vi "Counter - Read Encoder.vi"() -> ()   [LabVIEW 2022 SP3]
doc: "This example demonstrates how to use a counter to continually monitor the angular position of an encoder.\n\nFor instructions on how to connect your signals to the DAQ device, refer to your device documentation."
uses:
  <vilib>/Utility/error.llb/DialogType.ctl
  <vilib>/DAQmx/read.llb/DAQmx Read (Counter DBL 1Chan 1Samp).vi
  <vilib>/DAQmx/create/channels.llb/DAQmx Create Channel (CI-Position-Angular Encoder).vi
  <vilib>/DAQmx/miscellaneous.llb/DAQmx Fill In Error Info.vi
  <resource>/objmgr/daqmx.rc
panel:
  in  "Z Index Terminal":tag="PFI9"
  in  "Z Index Enable":bool
  in  "Pulses Per Revolution":u32=24
  in  "B Input Terminal":tag="PFI10"
  out "Position":dbl
  in  "A Input Terminal":tag="PFI8"
  in  "Counter":tag="Dev1/ctr0"
  in  "Trigger Type":enum32{"No Trigger", "Digital Arm Start"}(tab)
  in  "Edge":i32(ring)=10280 items=["Rising"=10280, "Falling"=10171]
  in  "Digital Trigger Source":tag
  in  "Stop":bool
  in  "Loop Time (ms)":u32=10
  # "Channel Settings"
  # "Acquired Data"
  # "Timing Settings"
  # "Trigger Settings"
  # "To configure and use a trigger or the count reset you must have the necessary tab selected above.  Not all hardware supports the above options--refer to your device documentation for more info."
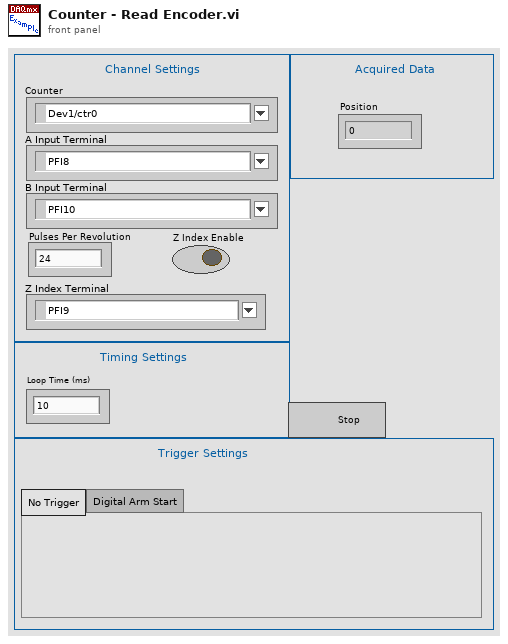
[diagram p1: front panel]
types:
  T1 = typedef "DialogType.ctl" = u16
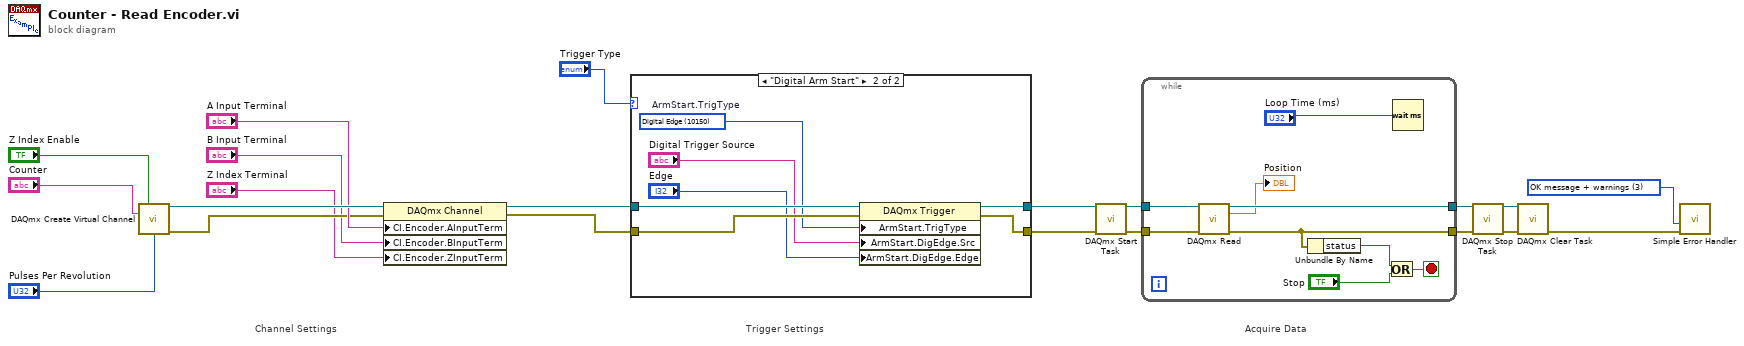
[diagram p0: block diagram]
diagram:
  w1 = T1 3 items=["no dialog", "OK message", "continue or stop message", "OK message + warnings", "continue/stop + warnings"] ("type of dialog (OK msg:1)")
  # "Acquire Data"
  # "Trigger Settings"
  # "Channel Settings"
  n1 = call-poly <vilib>:"DAQmx Create Virtual Channel.vi"("z index enable"="Z Index Enable", "counter"="Counter", "pulses per revolution"="Pulses Per Revolution") -> ("task out"=w14:refnum<k21>, "error out"=w12:errorcluster)  [unwired: 11 in]
  n2 = property class="DAQmx Channel"(reference=w14, error in=w12, "CI.Encoder.AInputTerm"="A Input Terminal", "CI.Encoder.BInputTerm"="B Input Terminal", "CI.Encoder.ZInputTerm"="Z Index Terminal") -> (reference out=w10:refnum<k21>, error out=w11:errorcluster)
  n3 = case shown="\"Digital Arm Start\"" "Trigger Type" {
    tunnel: w10 -> [w23 w30]
    tunnel: w11 -> [w22 w27]
    tunnel: [w23 w29] -> w21
    tunnel: [w22 w28] -> w20
    frame "No Trigger", Default {
    }
    frame "Digital Arm Start" {
      w24 = 10150 items=["Digital Edge"=10150, "None"=10230]  # ArmStart.TrigType
      n4 = property class="DAQmx Trigger"(reference=w30, error in=w27, "ArmStart.TrigType"=w24, "ArmStart.DigEdge.Src"="Digital Trigger Source", "ArmStart.DigEdge.Edge"="Edge") -> (reference out=w29:refnum<k21>, error out=w28:errorcluster)
    }
  }
  n5 = call <vilib>:"DAQmx Start Task.vi"("task/channels in"=w21, "error in"=w20) -> ("task out"=w19:refnum<k21>, "error out"=w18:errorcluster)  [unwired: 12 in]
  n6 = while {
    tunnel: w19 -> [w39]
    tunnel: w18 -> [w38]
    tunnel: [w35] -> w4
    tunnel: [w36] -> w5
    stop <- w37 stop-if-true
    n7 = call-poly <vilib>:"DAQmx Read.vi"("task/channels in"=w39, "error in"=w38) -> ("task out"=w36:refnum<k21>, "data"=→"Position":dbl, "error out"=w35:errorcluster)  [unwired: 11 in]
    n8 = Unbundle By Name(w35) -> ("status"=w34:bool)
    n9 = Or(x=w34, y="Stop") -> (x .or. y?=w37:bool)
    n10 = Wait (ms)(milliseconds to wait="Loop Time (ms)") -> ()  [unwired: 1 out]
  }
  n11 = call <vilib>:"DAQmx Stop Task.vi"("task/channels in"=w5, "error in"=w4) -> ("task out"=w2:refnum<k21>, "error out"=w3:errorcluster)  [unwired: 12 in]
  n12 = call <vilib>:"DAQmx Clear Task.vi"("task in"=w2, "error in"=w3) -> ("error out"=w17:errorcluster)  [unwired: 13 in]
  n13 = call <vilib>:"Simple Error Handler.vi"("type of dialog (OK msg:1)"=w1, "error in (no error)"=w17) -> ()  [unwired: 3 in, 5 out]
